vi "Box-Muller.vi"(10 "sigma":dbl, 11 "mu":dbl) -> (3 "x":dbl)   [LabVIEW 2017]
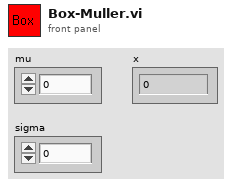
[diagram p1: front panel]
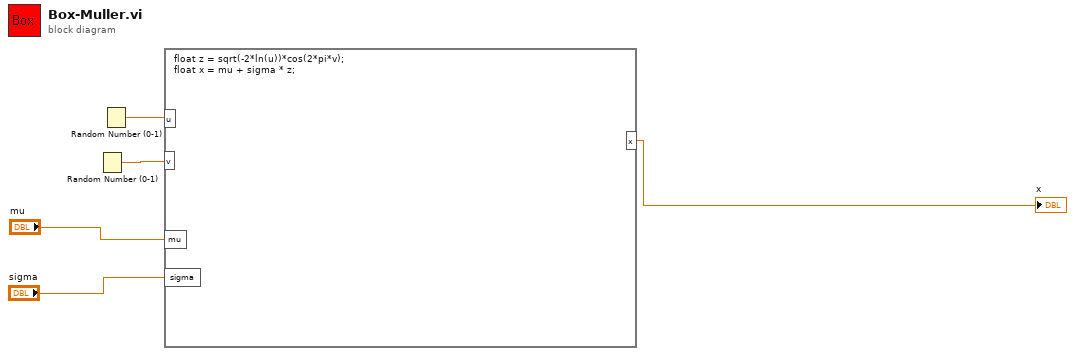
[diagram p0: block diagram]
diagram:
  n1 = Random Number (0-1)() -> (number: 0 to 1=w2:dbl)
  n2 = Random Number (0-1)() -> (number: 0 to 1=w1:dbl)
  n3 = formula code="float z = sqrt(-2*ln(u))*cos(2*pi*v);\nfloat x = mu + sigma * z;"("u"=w1, "v"=w2, "mu"="mu", "sigma"="sigma") -> ("x"=→"x":dbl)
